vi "AddFolder.vi"(7 "folder_node":string, 8 "error in (no error)":errorcluster, 9 "folder_browse":string, 10 "folder_display":string, 11 "Server in":refnum<class "Server.lvclass">) -> (0 "error out":errorcluster, 3 "Server out":refnum<class "Server.lvclass">)   [LabVIEW 2017, in "opcua.lvlib" / "Server.lvclass"]
uses:
  Server.lvclass
  Server.lvclass/Server.ctl
  opcua32.dll
  opcua.lvlib
panel:
  in  "ns":i32=2
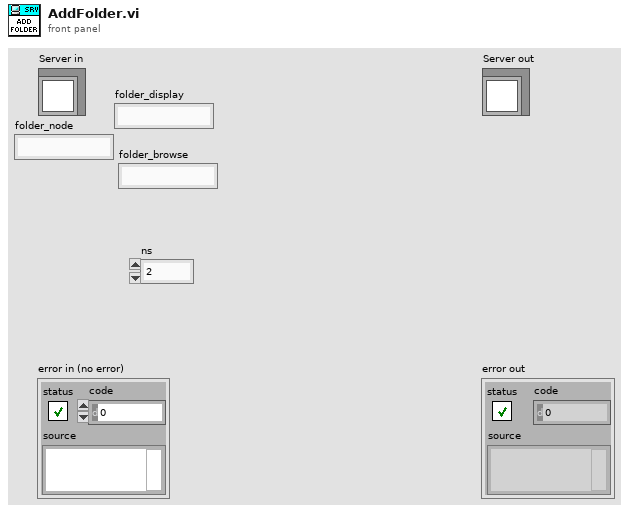
[diagram p1: front panel]
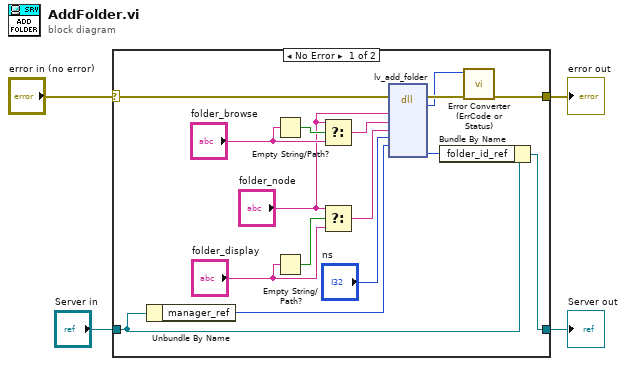
[diagram p0: block diagram]
diagram:
  n1 = case shown="No Error" "error in (no error)" {
    selector: "error in (no error)" -> [w19 w21]
    tunnel: [w6 w21] -> w3
    tunnel: [w16 w22] -> w1
    tunnel: "Server in" -> [w17 w22]
    frame No Error {
      n2 = Unbundle By Name(w17) -> ("manager_ref"=w20:u64)
      n3 = Empty String/Path?(string/path="folder_browse") -> (empty?=w14:bool)
      n4 = Empty String/Path?(string/path="folder_display") -> (empty?=w11:bool)
      n5 = Select(t="folder_node", s=w14, f="folder_browse") -> (s? t:f=w12:string)
      n6 = Select(t="folder_node", s=w11, f="folder_display") -> (s? t:f=w8:string)
      n7 = dll-call lib="C:/Users/Andrey/Desktop/opcua-labview/opcua-lvlib/opcua*.dll" fn="lv_add_folder"(error in=w19, "folder_node"="folder_node", "folder_browse"=w12, "folder_display"=w8, "ns"="ns", "manager"=w20) -> (error out=w7:errorcluster, "return type"=w5:i32, "folder_id_out"=w15:u64)  [unwired: 8 in, 1 out]
      n8 = Bundle By Name(cluster=w17, "folder_id_ref"=w15) -> (w16:refnum<class "Server.lvclass">)
      n9 = call "Error Converter (ErrCode or Status).vi"("error in (no error)"=w7, "error code"=w5) -> ("error out"=w6:errorcluster)  [unwired: 9 in]
    }
    frame Error {
    }
  }
  "error out" <- w3
  "Server out" <- w1
